vi "示例 4.vi"() -> ()   [LabVIEW 2021]
uses:
  <vilib>/measure/NI_MABase.lvlib
panel:
  in  "stop":bool
  out "波形图":waveform(dbl)(graph)
  in  "波形":enum16{"锯齿", "正弦", "方波", "三角"}(ring)
  in  "振幅":dbl
  in  "频率":dbl
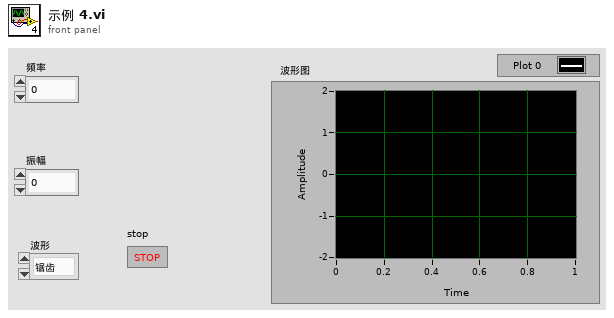
[diagram p1: front panel]
types:
  T1 = enum16{"Sine Wave", "Triangle Wave", "Square Wave", "Sawtooth Wave"}
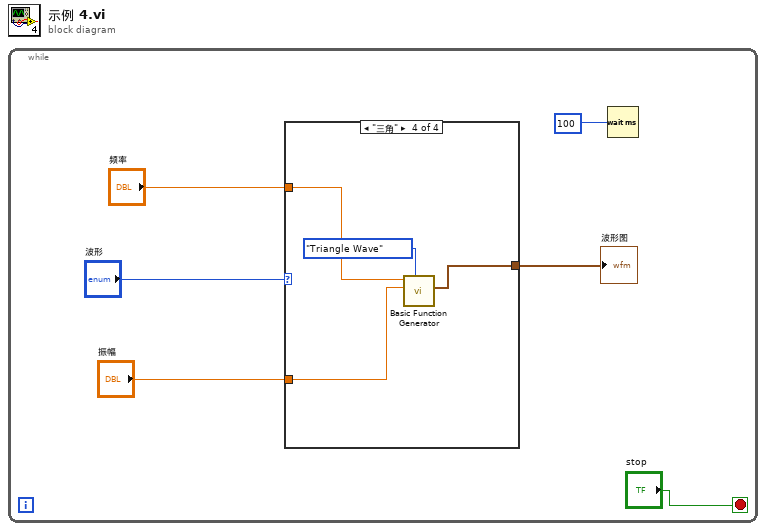
[diagram p0: block diagram]
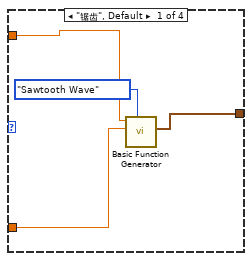
[diagram p2: hidden frame]
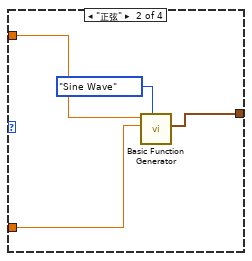
[diagram p3: hidden frame]
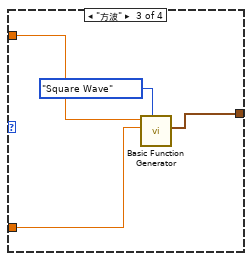
[diagram p4: hidden frame]
diagram:
  n1 = while {
    stop <- "stop" stop-if-true
    n2 = case shown="\"三角\"" "波形" {
      tunnel: "频率" -> [w10 w14 w18 w22]
      tunnel: "振幅" -> [w9 w13 w17 w21]
      tunnel: [w8 w12 w15 w19] -> w3
      frame "锯齿", Default {
        n3 = call <vilib>:"Basic Function Generator.vi"("signal type"=T1."Sawtooth Wave", "amplitude"=w9, "frequency"=w10) -> ("signal out"=w8:waveform(dbl))  [unwired: 6 in, 2 out]
      }
      frame "正弦" {
        n4 = call <vilib>:"Basic Function Generator.vi"("signal type"=T1."Sine Wave", "amplitude"=w13, "frequency"=w14) -> ("signal out"=w12:waveform(dbl))  [unwired: 6 in, 2 out]
      }
      frame "方波" {
        n5 = call <vilib>:"Basic Function Generator.vi"("signal type"=T1."Square Wave", "amplitude"=w17, "frequency"=w18) -> ("signal out"=w15:waveform(dbl))  [unwired: 6 in, 2 out]
      }
      frame "三角" {
        n6 = call <vilib>:"Basic Function Generator.vi"("signal type"=T1."Triangle Wave", "amplitude"=w21, "frequency"=w22) -> ("signal out"=w19:waveform(dbl))  [unwired: 6 in, 2 out]
      }
    }
    "波形图" <- w3
    n7 = Wait (ms)(milliseconds to wait=100) -> ()  [unwired: 1 out]
  }
